vi "WaitForMapUpdate.vi"(9 "Error In":errorcluster, 10 "Map":refnum<k7>) -> (2 "Error Out":errorcluster, 3 "Map Out":refnum<k7>)   [LabVIEW 2010]
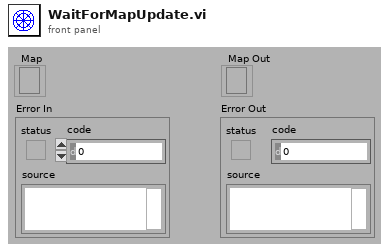
[diagram p1: front panel]
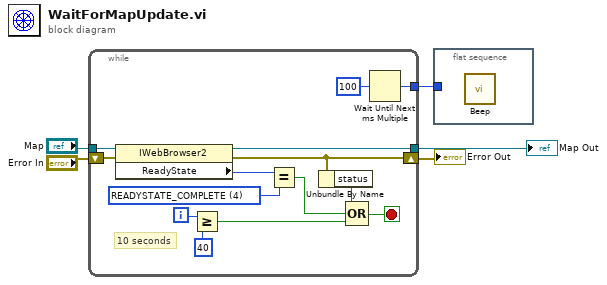
[diagram p0: block diagram]
diagram:
  n1 = while {
    tunnel: "Map" -> [w19]
    shift-right: [w15] -> w4
    shift-left: "Error In" -> [w18]
    tunnel: [w7] -> w5
    tunnel: [w6] -> w1
    i -> [w13]
    stop <- w8 stop-if-true
    w16 = 4 items=["READYSTATE_UNINITIALIZED", "READYSTATE_LOADING", "READYSTATE_LOADED", "READYSTATE_INTERACTIVE", "READYSTATE_COMPLETE"] ("ReadyState")
    # "10 seconds"
    n2 = property class="IWebBrowser2"(reference=w19, error in=w18) -> (reference out=w6:refnum<k7>, error out=w15:errorcluster, "ReadyState"=w17:i32)
    n3 = Greater Or Equal?(x=w13, y=40) -> (x >= y?=w9:bool)
    n4 = Equal?(x=w17, y=w16) -> (x = y?=w10:bool)
    n5 = Unbundle By Name(w15) -> ("status"=w11:bool)
    n6 = Compound Arithmetic op=OR(w11, w10, w9) -> (w8:bool)
    n7 = Wait Until Next ms Multiple(millisecond multiple=u32 100) -> (millisecond timer value=w7:u32)
  }
  "Error Out" <- w4
  "Map Out" <- w1
  n8 = flat-sequence {
    tunnel: w5 -> [_]
    frame #0 {
      n9 = call <vilib>:"Beep.vi"() -> ()  [unwired: 12 in]
    }
  }
